vi "Initialize save file.vi"(4 "Number of samples per channel":i32, 6 "Sampling rate":dbl, 8 "error in (no error)":errorcluster, 9 "Headers":string[](array[string])=["Time (s)", "Voltage1 (kV)", "Voltage2 (kV)", "Current1 (uA)", "Current2 (uA)", "VoltDiv1 (V)", "VoltDiv2 (V)"], 10 "Save data? in":bool, 11 "Save data path in":path) -> (0 "error out":errorcluster, 2 "Save data? out":bool, 3 "Save data path out":path)   [LabVIEW 2018]
uses:
  <vilib>/Utility/file.llb/Write Delimited Spreadsheet (string).vi
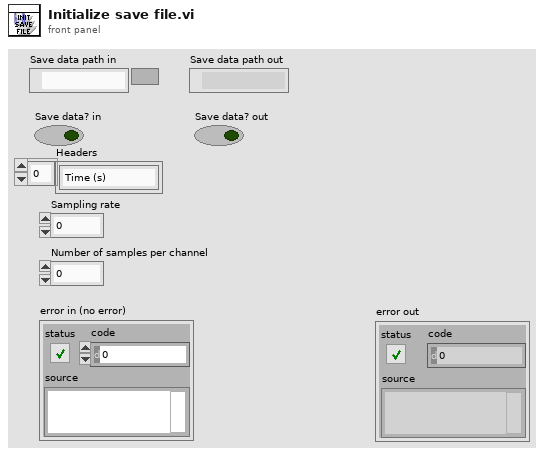
[diagram p1: front panel]
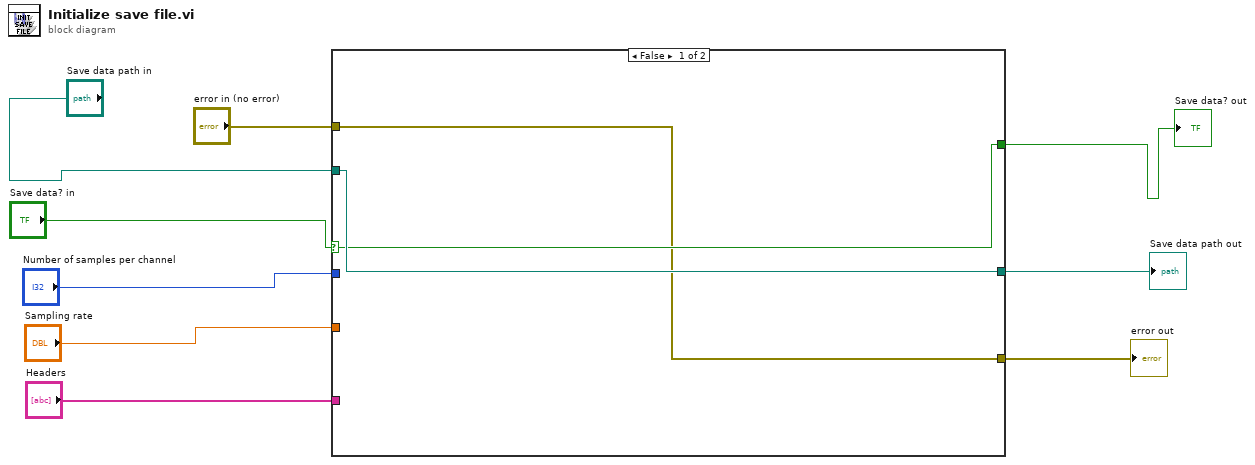
[diagram p0: block diagram]
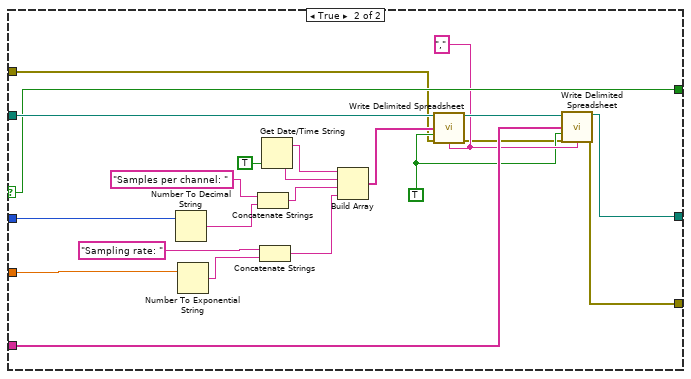
[diagram p2: hidden frame]
diagram:
  n1 = case shown="False" "Save data? in" {
    selector: "Save data? in" -> [w11 w18]
    tunnel: "Save data path in" -> [w12 w23]
    tunnel: "Sampling rate" -> [_ w22]
    tunnel: "Number of samples per channel" -> [_ w21]
    tunnel: "Headers" -> [_ w20]
    tunnel: [w12 w19] -> w5
    tunnel: [w11 w18] -> w3
    tunnel: [w10 w14] -> w2
    tunnel: "error in (no error)" -> [w10 w13]
    frame False {
    }
    frame True {
      w17 = "," ("delimiter (Tab)")
      w16 = TRUE ("append to file? (new file:F)")
      n2 = Number To Decimal String(number=w21) -> (decimal integer string=w34:string)  [unwired: 1 in]
      n3 = Number To Exponential String(number=w22) -> (E-format string=w32:string)  [unwired: 3 in]
      n4 = Concatenate Strings("Samples per channel: " ("string"), w34) -> (w30:string)
      n5 = Concatenate Strings("Sampling rate: " ("string"), w32) -> (w29:string)
      n6 = Get Date/Time String(want seconds? (F)=TRUE) -> (date string=w28:string, time string=w27:string)  [unwired: 2 in]
      n7 = Build Array(w28, w27, w30, w29) -> (w26:string[])
      n8 = call-poly <vilib>:"Write Delimited Spreadsheet.vi"("file path (dialog if empty)"=w23, "1D data"=w26, "append to file? (new file:F)"=w16, "error in (no error)"=w13, "delimiter (\\t)"=w17) -> ("new file path (Not A Path if cancelled)"=w24:path, "error out"=w15:errorcluster)  [unwired: 9 in]
      n9 = call-poly <vilib>:"Write Delimited Spreadsheet.vi"("file path (dialog if empty)"=w24, "1D data"=w20, "append to file? (new file:F)"=w16, "error in (no error)"=w15, "delimiter (\\t)"=w17) -> ("new file path (Not A Path if cancelled)"=w19:path, "error out"=w14:errorcluster)  [unwired: 9 in]
    }
  }
  "Save data path out" <- w5
  "Save data? out" <- w3
  "error out" <- w2
